vi "Focuser JSON to cluster.vi"(11 "JSON status":string) -> (3 "Focuser160":T3={"absolute"=FALSE, "alarm"=FALSE, "broker"="", "cmd"={"clientId"=0.0, "clientTransactionId"=0.0, "clientName"="", "action"="\n     }"}, "connected"=FALSE, "controller"="", "device"="", "error"="", "homing"=FALSE, "initialized"=FALSE, "isMoving"=FALSE, "maxSpeed"=0.0, "maxStep"=0.0, "position"=0.0, "tempComp"=FALSE, "tempCompAvailable"=FALSE, "temperature"=0.0, "timestamp"="", "version"=""})   [LabVIEW 2012]
panel:
  in  "focuserNoCmd":T1
  in  "cmdAlone":T2={"clientId"=0.0, "clientTransactionId"=0.0, "clientName"="", "action"="\n     }"}
  # "O nome e o tipo de dados dos\ncontroles do indicador \"JSON cluster\" devem ser iguais aos \nkeywords e valores da string \"JSON status\"."
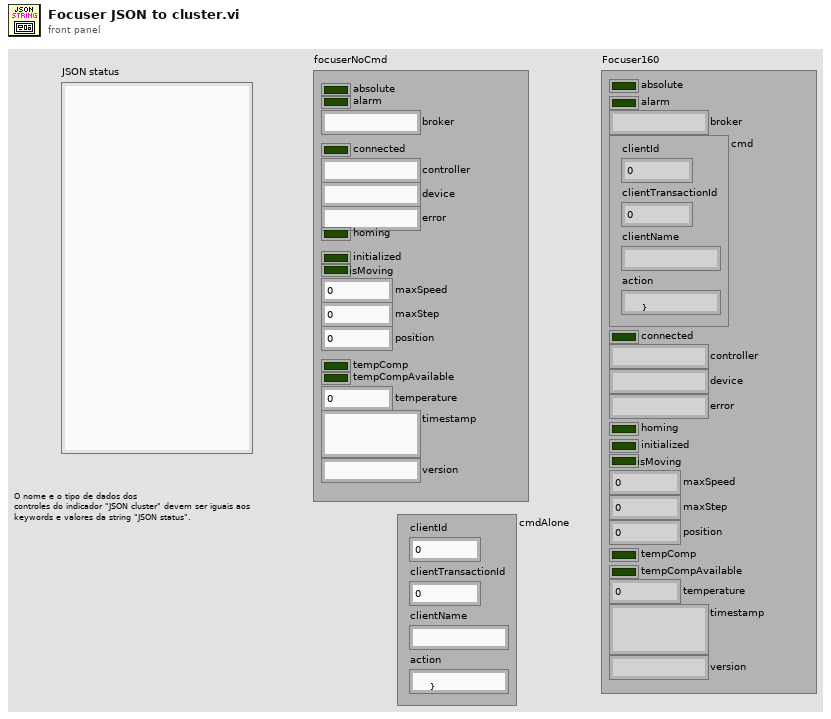
[diagram p1: front panel]
types:
  T1 = cluster{"absolute":bool, "alarm":bool, "broker":string, "connected":bool, "controller":string, "device":string, "error":string, "homing":bool, "initialized":bool, "isMoving":bool, "maxSpeed":dbl, "maxStep":dbl, "position":dbl, "tempComp":bool, "tempCompAvailable":bool, "temperature":dbl, "timestamp":string, "version":string}
  T2 = cluster{"clientId":dbl, "clientTransactionId":dbl, "clientName":string, "action":string}
  T3 = cluster{"absolute":bool, "alarm":bool, "broker":string, "cmd":cluster{"clientId":dbl, "clientTransactionId":dbl, "clientName":string, "action":string}, "connected":bool, "controller":string, "device":string, "error":string, "homing":bool, "initialized":bool, "isMoving":bool, "maxSpeed":dbl, "maxStep":dbl, "position":dbl, "tempComp":bool, "tempCompAvailable":bool, "temperature":dbl, "timestamp":string, "version":string}
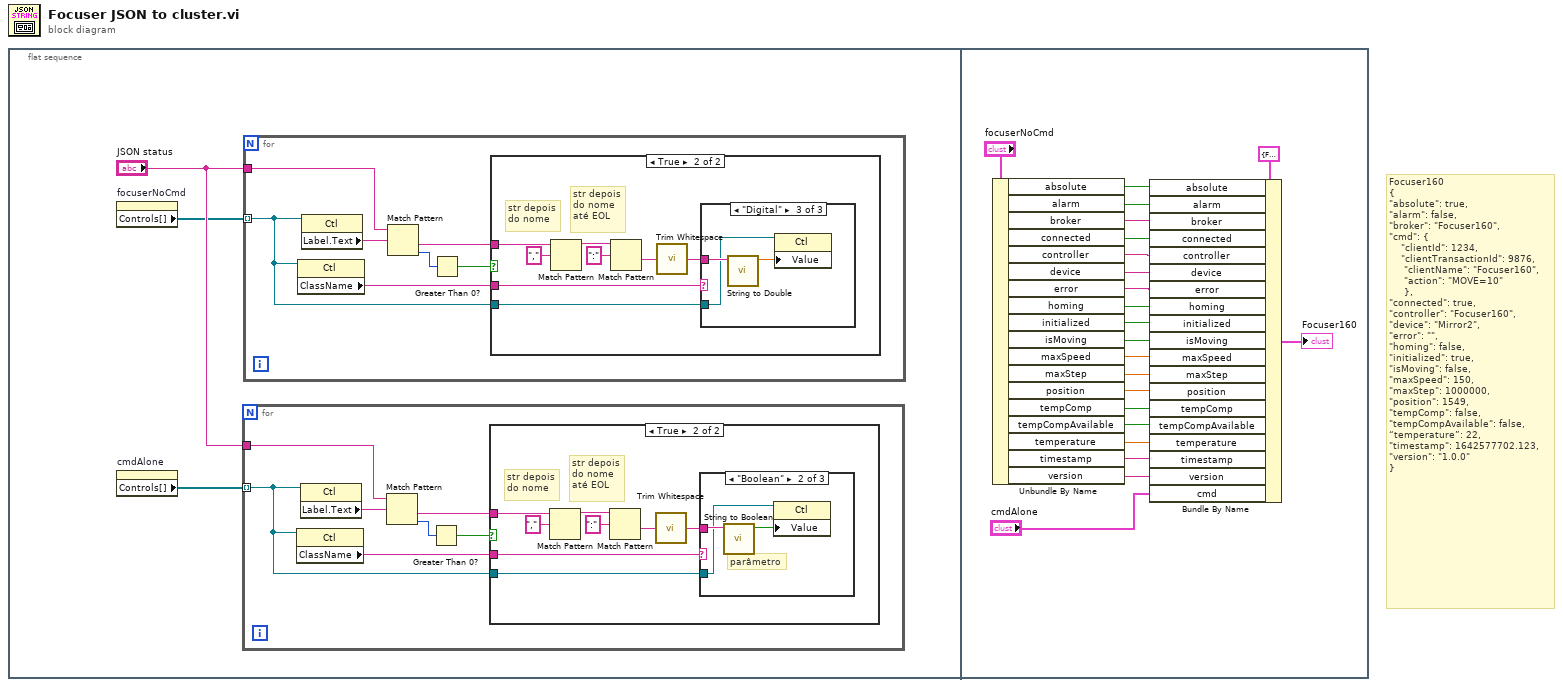
[diagram p0: block diagram]
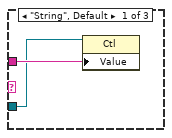
[diagram p3: hidden frame]
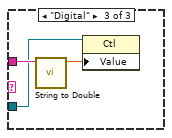
[diagram p4: hidden frame]
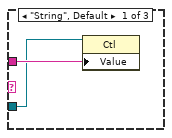
[diagram p6: hidden frame]
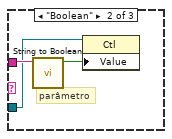
[diagram p7: hidden frame]
diagram:
  # "Focuser160\n{\n\"absolute\": true,\n\"alarm\": false,\n\"broker\": \"Focuser160\",\n\"cmd\": {\n    \"clientId\": 1234,\n    \"clientTransactionId\": 9876,\n     \"clientName\": \"Focuser160\",\n     \"action\": \"MOVE=10\"\n     },\n\"connected\": true,\n\"controller\": \"Focuser160\",\n\"device\": \"Mirror2\",\n\"error\": \"\",\n\"homing\": false,\n\"initialized\": true,\n\"isMoving\": false,\n\"maxSpeed\": 150,\n\"maxStep\": 1000000,\n\"position\": 1549,\n\"tempComp\": false,\n\"tempCompAvailable\": false,\n“temperature”: 22,\n\"timestamp\": 1642577702.123,\n\"version\": \"1.0.0\"\n}"
  n1 = flat-sequence {
    frame #0 {
      n2 = property on="focuserNoCmd" class="Clust (strict)"() -> ("Controls[]"=w1:refnum<vi>[])  [unwired: 2 in, 2 out]
      n3 = property on="cmdAlone" class="Clust (strict)"() -> ("Controls[]"=w3:refnum<vi>[])  [unwired: 2 in, 2 out]
      n4 = for {
        tunnel: w3 -> [w4] mode=indexing
        tunnel: "JSON status" -> [w7]
        n5 = property class="Ctl"(reference=w4) -> ("ClassName"=w5:string)  [unwired: 1 in, 2 out]
        n6 = property class="Ctl"(reference=w4) -> ("Label.Text"=w10:string)  [unwired: 1 in, 2 out]
        n7 = Match Pattern(string=w7, regular expression=w10) -> (after substring=w6:string, offset past match=w9:i32)  [unwired: 1 in, 2 out]
        n8 = Greater Than 0?(x=w9) -> (x > 0?=w8:bool)
        n9 = case shown="True" w8 {
          tunnel: w6 -> [_ w18]
          tunnel: w5 -> [_ w14]
          tunnel: w4 -> [_ w13]
          frame False {
          }
          frame True {
            # "str depois\ndo nome\naté EOL"
            # "str depois\ndo nome"
            n10 = Match Pattern(string=w18, regular expression=",") -> (before substring=w16:string)  [unwired: 1 in, 3 out]
            n11 = Match Pattern(string=w16, regular expression=":") -> (after substring=w11:string)  [unwired: 1 in, 3 out]
            n12 = call <vilib>:"Trim Whitespace.vi"("string"=w11) -> ("trimmed string"=w12:string)  [unwired: 1 in]
            n13 = case shown="\"Boolean\"" w14 {
              tunnel: w12 -> [w20 w23 w26]
              tunnel: w13 -> [w19 w22 w25]
              frame "String", Default {
                n14 = property class="Ctl"(reference=w19, "Value"=w20) -> ()  [unwired: 1 in, 2 out]
              }
              frame "Boolean" {
                # "parâmetro"
                n15 = call "String to Boolean.vi"("booleanString"=w23) -> ("state"=w21:bool)  [unwired: 10 in]
                n16 = property class="Ctl"(reference=w22, "Value"=w21) -> ()  [unwired: 1 in, 2 out]
              }
              frame "Digital" {
                n17 = call "String to Double.vi"("fractionalString"=w26) -> ("value"=w24:dbl)  [unwired: 10 in]
                n18 = property class="Ctl"(reference=w25, "Value"=w24) -> ()  [unwired: 1 in, 2 out]
              }
            }
          }
        }
      }
      n19 = for {
        tunnel: w1 -> [w27] mode=indexing
        tunnel: "JSON status" -> [w30]
        n20 = property class="Ctl"(reference=w27) -> ("ClassName"=w28:string)  [unwired: 1 in, 2 out]
        n21 = property class="Ctl"(reference=w27) -> ("Label.Text"=w33:string)  [unwired: 1 in, 2 out]
        n22 = Match Pattern(string=w30, regular expression=w33) -> (after substring=w29:string, offset past match=w32:i32)  [unwired: 1 in, 2 out]
        n23 = Greater Than 0?(x=w32) -> (x > 0?=w31:bool)
        n24 = case shown="True" w31 {
          tunnel: w29 -> [_ w41]
          tunnel: w28 -> [_ w37]
          tunnel: w27 -> [_ w36]
          frame False {
          }
          frame True {
            # "str depois\ndo nome\naté EOL"
            # "str depois\ndo nome"
            n25 = Match Pattern(string=w41, regular expression=",") -> (before substring=w39:string)  [unwired: 1 in, 3 out]
            n26 = Match Pattern(string=w39, regular expression=":") -> (after substring=w34:string)  [unwired: 1 in, 3 out]
            n27 = call <vilib>:"Trim Whitespace.vi"("string"=w34) -> ("trimmed string"=w35:string)  [unwired: 1 in]
            n28 = case shown="\"Digital\"" w37 {
              tunnel: w35 -> [w43 w46 w49]
              tunnel: w36 -> [w42 w45 w48]
              frame "String", Default {
                n29 = property class="Ctl"(reference=w42, "Value"=w43) -> ()  [unwired: 1 in, 2 out]
              }
              frame "Boolean" {
                # "parâmetro"
                n30 = call "String to Boolean.vi"("booleanString"=w46) -> ("state"=w44:bool)  [unwired: 10 in]
                n31 = property class="Ctl"(reference=w45, "Value"=w44) -> ()  [unwired: 1 in, 2 out]
              }
              frame "Digital" {
                n32 = call "String to Double.vi"("fractionalString"=w49) -> ("value"=w47:dbl)  [unwired: 10 in]
                n33 = property class="Ctl"(reference=w48, "Value"=w47) -> ()  [unwired: 1 in, 2 out]
              }
            }
          }
        }
      }
    }
    frame #1 {
      n34 = Unbundle By Name("focuserNoCmd") -> ("absolute"=w67:bool, "alarm"=w66:bool, "broker"=w65:string, "connected"=w64:bool, "controller"=w63:string, "device"=w62:string, "error"=w61:string, "homing"=w60:bool, "initialized"=w59:bool, "isMoving"=w58:bool, "maxSpeed"=w57:dbl, "maxStep"=w56:dbl, "position"=w55:dbl, "tempComp"=w54:bool, "tempCompAvailable"=w53:bool, "temperature"=w52:dbl, "timestamp"=w51:string, "version"=w50:string)
      n35 = Bundle By Name(cluster=T3 {"absolute"=FALSE, "alarm"=FALSE, "broker"="", "cmd"={"clientId"=0.0, "clientTransactionId"=0.0, "clientName"="", "action"="\n     }"}, "connected"=FALSE, "controller"="", "device"="", "error"="", "homing"=FALSE, "initialized"=FALSE, "isMoving"=FALSE, "maxSpeed"=0.0, "maxStep"=0.0, "position"=0.0, "tempComp"=FALSE, "tempCompAvailable"=FALSE, "temperature"=0.0, "timestamp"="", "version"=""} ("Focuser160"), "absolute"=w67, "alarm"=w66, "broker"=w65, "connected"=w64, "controller"=w63, "device"=w62, "error"=w61, "homing"=w60, "initialized"=w59, "isMoving"=w58, "maxSpeed"=w57, "maxStep"=w56, "position"=w55, "tempComp"=w54, "tempCompAvailable"=w53, "temperature"=w52, "timestamp"=w51, "version"=w50, "cmd"="cmdAlone") -> (→"Focuser160":T3)
    }
  }
